vi "CRYNew Directory to Tree.vi"(6 "pattern":string, 8 "error in":errorcluster, 9 "Parent Tag":string, 10 "directory path":path, 11 "Tree":refnum<vi>) -> (0 "error out":errorcluster, 3 "Tree":refnum<vi>)   [LabVIEW 2013]
doc: "This subVI populates the tree control with information obtained from the directory you specify in the directory path field."
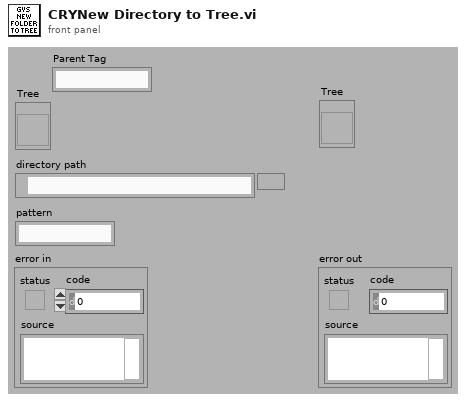
[diagram p1: front panel]
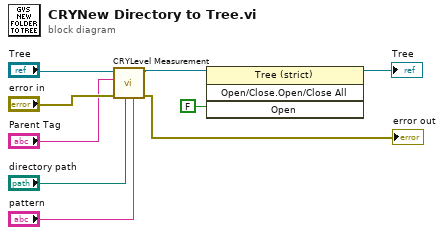
[diagram p0: block diagram]
diagram:
  n1 = call "CRYLevel Measurement.vi"("pattern"="pattern", "directory path"="directory path", "error in"="error in", "Parent Tag"="Parent Tag", "Tree In"="Tree") -> ("error out"=→"error out":errorcluster, "Tree Out"=w1:refnum<vi>)  [unwired: 5 in]
  n2 = invoke on="Invoke Node" class="Tree (strict)" method="Open/Close.Open/Close All"(reference=w1, "Open"=FALSE) -> (reference out=→"Tree":refnum<vi>)  [unwired: 2 in, 3 out]
